vi "Date Time String to time stamp.vi"(8 "error in (no error)":errorcluster, 11 "Sample Date Time String":string) -> (0 "error out":errorcluster, 3 "Timestamp from Number of Seconds":timestamp)   [LabVIEW 2024]
doc: "This example is used to convert a date and time string back into a timestamp."
uses:
  <vilib>/Utility/miscctls.llb/LVDateTimeRec.ctl
panel:
  out "Number of Seconds":u64
  out "Timestamp from Date/Time String":timestamp
  # "Derived/Computed Values"
  # "Note: the only thing that's off is the Fractional Seconds, but that's because you don't have that information\nin the date/time string"
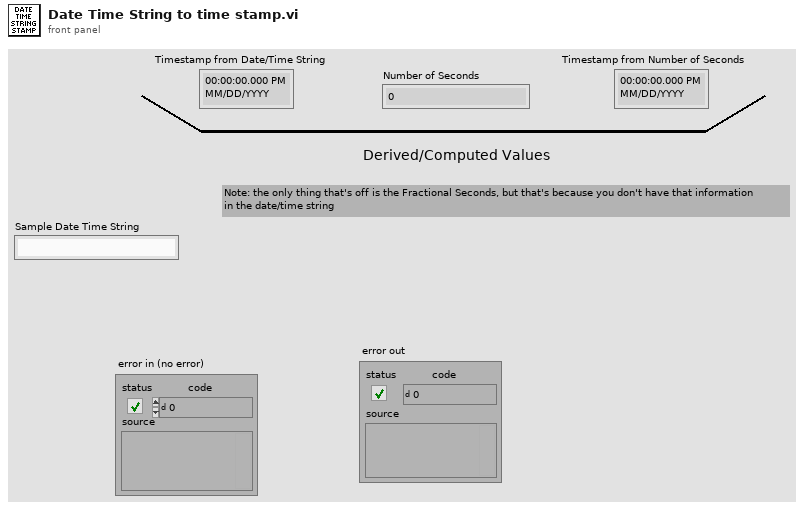
[diagram p1: front panel]
types:
  T1 = typedef "LVDateTimeRec.ctl" = cluster{"fractional second":dbl, "second":i32, "minute":i32, "hour":i32, "day of month":i32, "month":i32, "year":i32, "day of week":i32, "day of year":i32, "DST":i32}
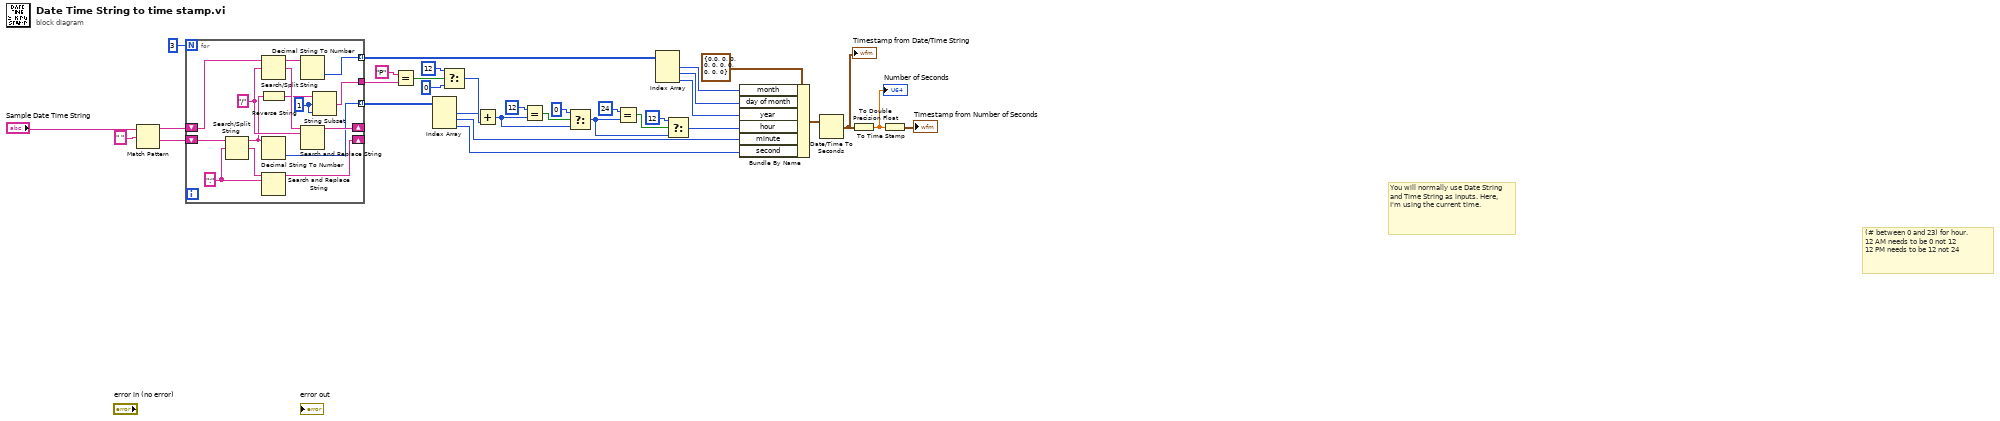
[diagram p0: block diagram]
diagram:
  # "You will normally use Date String and Time String as inputs. Here, I'm using the current time."
  # "(# between 0 and 23) for hour.\n12 AM needs to be 0 not 12\n12 PM needs to be 12 not 24"
  n1 = Match Pattern(string="Sample Date Time String", regular expression=" ") -> (before substring=w2:string, after substring=w1:string)  [unwired: 1 in, 2 out]
  n2 = for {
    N: 3 -> [_]
    shift-right: [w46] -> _
    shift-left: w2 -> [w47]
    tunnel: [w44] -> w23 mode=indexing
    shift-right: [w43] -> _
    shift-left: w1 -> [w39]
    tunnel: [w40] -> w30 mode=indexing
    tunnel: [w34] -> w32
    w35 = 1 ("offset (0)")
    w41 = ":" ("search string/char (-)")
    w42 = "/" ("search string/char (-)")
    n3 = Search/Split String(string=w39, search string/char (-)=w41) -> (substring before match=w37:string, match + rest of string=w38:string)  [unwired: 1 in, 1 out]
    n4 = Search/Split String(string=w47, search string/char (-)=w42) -> (substring before match=w45:string, match + rest of string=w48:string)  [unwired: 1 in, 1 out]
    n5 = Reverse String(1:w37) -> (0:w36:string)
    n6 = Decimal String To Number(string=w37) -> (number=w40:i32)  [unwired: 2 in, 1 out]
    n7 = Search and Replace String(input string=w38, search string=w41) -> (result string=w43:string)  [unwired: 6 in, 3 out]
    n8 = Decimal String To Number(string=w45) -> (number=w44:i32)  [unwired: 2 in, 1 out]
    n9 = Search and Replace String(input string=w48, search string=w42) -> (result string=w46:string)  [unwired: 6 in, 3 out]
    n10 = String Subset(string=w36, offset (0)=w35, length (rest)=w35) -> (substring=w34:string)
  }
  n11 = Equal?(x="P", y=w32) -> (x = y?=w29:bool)
  n12 = Index Array(array=w30) -> (element #1=w25:i32, element #2=w19:i32, element #3=w18:i32)  [unwired: 3 in]
  n13 = Select(t=12 ("index"), s=w29, f=0 ("index")) -> (s? t:f=w26:i32)
  n14 = Add(x=w25, y=w26) -> (x+y=w12:i32)
  n15 = Equal?(x=12 ("y"), y=w12) -> (x = y?=w14:bool)
  n16 = Select(t=0, s=w14, f=w12) -> (s? t:f=w9:i32)
  n17 = Equal?(x=24 ("y"), y=w9) -> (x = y?=w16:bool)
  n18 = Index Array(array=w23) -> (element #1=w22:i32, element #2=w21:i32, element #3=w20:i32)  [unwired: 3 in]
  n19 = Select(t=12 ("index"), s=w16, f=w9) -> (s? t:f=w8:i32)
  n20 = Bundle By Name(cluster=T1 {"fractional second"=0.0, "second"=0, "minute"=0, "hour"=0, "day of month"=0, "month"=0, "year"=0, "day of week"=0, "day of year"=0, "DST"=0} ("date time rec"), "month"=w22, "day of month"=w21, "year"=w20, "hour"=w8, "minute"=w19, "second"=w18) -> (w17:T1)
  n21 = Date/Time To Seconds(2:w17) -> (0:w7:timestamp)  [unwired: 1 in]
  "Timestamp from Date/Time String" <- w7
  n22 = To Double Precision Float(number=w7) -> (double precision float=w6:dbl)
  "Number of Seconds" <- w6
  n23 = To Time Stamp(1:w6) -> (0:→"Timestamp from Number of Seconds":timestamp)
